vi "GRNF_Kraken.vi"(7 "RefNum Name":string="My Motor RefNum") -> (0 "Error":errorcluster, 3 "Device Reference":T1)   [LabVIEW 2023]
doc: "This VI loads a CTRE motor refnum on code boot and then stores it in memory so that the information does not have to be queried on subsequent loop cycles. This VI is configured for polymorphic use."
uses:
  <vilib>/Rock Robotics/WPI/ThirdParty/Phoenix6/DeviceReference.ctl
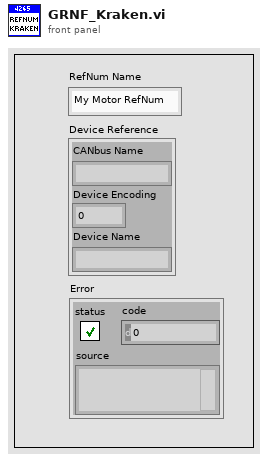
[diagram p1: front panel]
types:
  T1 = typedef "DeviceReference.ctl" = cluster{"CANbus Name":string, "Device Encoding":u32, "Device Name":string}
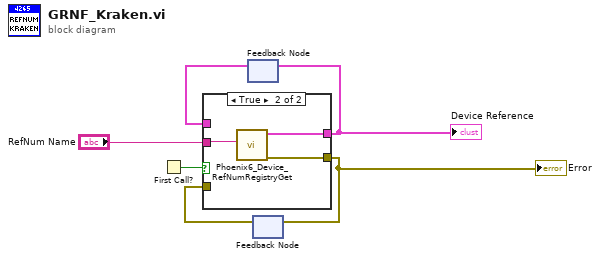
[diagram p0: block diagram]
diagram:
  n1 = First Call?() -> (First Call?: T/F=w6:bool)
  n2 = feedback #1() -> (w5:T1)  [unwired: 1 in]
  n3 = feedback #2() -> (w3:errorcluster)  [unwired: 1 in]
  n4 = case shown="True" w6 {
    tunnel: [w8 w11] -> w2
    tunnel: w5 -> [w8 _]
    tunnel: "RefNum Name" -> [_ w9]
    tunnel: [w7 w10] -> w1
    tunnel: w3 -> [w7 _]
    frame False {
    }
    frame True {
      n5 = call <vilib>:"Phoenix6_Device_RefNumRegistryGet.vi"("refnum name"=w9) -> ("error out"=w10:errorcluster, "data"=w11:T1)  [unwired: 9 in]
    }
  }
  "Error" <- w1
  "Device Reference" <- w2
  n6 = feedback-in #1(w2) -> ()
  n7 = feedback-in #2(w1) -> ()
